vi "ReadU64FromU16FIFO.vi"(1 "FIFO In":refnum<k21>="U16ResponseFIFO") -> (0 "U64":u64)   [LabVIEW 2016]
uses:
  <vilib>/rvi/DataTransferAndStorage/Container/Common/niFpgaContainerExecOnDevCompGetState.vi
  <vilib>/rvi/Emulation/niFpgaEmulationIsFPGAContextNoSignature.vi
  <vilib>/rvi/Emulation/niFpgaSctlEmulationGetInTimedLoop.vi
  <vilib>/rvi/errors/niFpgaSetErrorForExecOnDevCompSimple.vi
  <vilib>/rvi/eio/common/nirviEmuReportErrorAndStop.vi
  <vilib>/rvi/DataTransferAndStorage/Container/Common/niFpgaContainerGetUniqueNameForEmu.vi
  <vilib>/rvi/FIFO/Fifo_Resource/nirvififoEmulationSetSize.vi
  <vilib>/rvi/FIFO/Fifo_Resource/nirviFifoEmulationQueueMgr.vi
  <instcachedir>/0/nirviFifoEmulationQueueMgr_E5CAEC123FF24DC58D834DCA3CDAA9B5.lvgen/nirviFifoEmulationQueueMgr_E5CAEC123FF24DC58D834DCA3CDAA9B5_002.vi
  <vilib>/rvi/FIFO/Fifo_Resource/nirvififoEmulationDetermineInputValidOut.vi
  <vilib>/rvi/FIFO/Fifo_Resource/nirvififoEmulationCreateLock.vi
  <vilib>/rvi/Emulation/niFpgaProcessEmulError.vi
  <vilib>/rvi/FIFO/Fifo_Resource/nirvififoEmulationObtainLock.vi
  <vilib>/rvi/FIFO/Fifo_Resource/nirvififoEmulationReleaseLock.vi
  <vilib>/rvi/occurrence/nirviWaitOnOccurrenceBase.vi
  <vilib>/rvi/errors/nirviReportUnexpectedCaseInternalError.vi
  <vilib>/rvi/errors/nirviReportUnexpectedCaseInternalError (U32).vi
  <vilib>/Utility/error.llb/Clear Errors.vi
  <vilib>/rvi/interface/RandomDataEmulation/niFpgaRandomDataHandleErrors.vi
  <vilib>/rvi/DataTransferAndStorage/Container/XNode/niFpgaContainer.xnode
  <vilib>/rvi/FIFO/Fifo_Resource/niFpgaFifoEmulationRefIn.vi
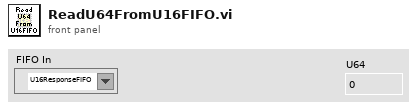
[diagram p1: front panel]
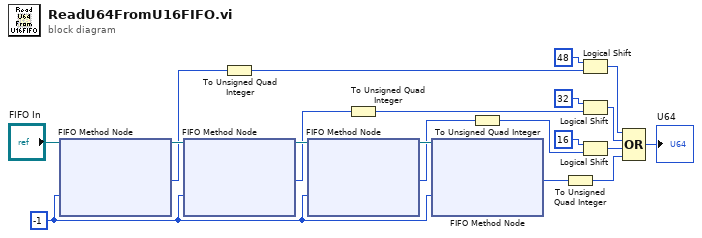
[diagram p0: block diagram]
diagram:
  w13 = -1 ("Timeout")
  n1 = xnode ("FIFO Method Node")("Timeout"=w13, "FIFO In"="FIFO In") -> ("Element"=w15:u16, "FIFO Out"=w19:refnum<k21>)  [unwired: 1 out]
  n2 = xnode ("FIFO Method Node")("Timeout"=w13, "FIFO In"=w19) -> ("Element"=w12:u16, "FIFO Out"=w18:refnum<k21>)  [unwired: 1 out]
  n3 = To Unsigned Quad Integer(1:w15) -> (0:w14:u64)
  n4 = xnode ("FIFO Method Node")("Timeout"=w13, "FIFO In"=w18) -> ("Element"=w11:u16, "FIFO Out"=w17:refnum<k21>)  [unwired: 1 out]
  n5 = To Unsigned Quad Integer(1:w12) -> (0:w9:u64)
  n6 = xnode ("FIFO Method Node")("Timeout"=w13, "FIFO In"=w17) -> ("Element"=w6:u16)  [unwired: 2 out]
  n7 = To Unsigned Quad Integer(1:w11) -> (0:w7:u64)
  n8 = To Unsigned Quad Integer(1:w6) -> (0:w2:u64)
  n9 = Logical Shift(y=i16 48, x=w14) -> (x << y=w5:u64)
  n10 = Logical Shift(y=i16 32, x=w9) -> (x << y=w4:u64)
  n11 = Logical Shift(y=i16 16, x=w7) -> (x << y=w3:u64)
  n12 = Compound Arithmetic op=OR(w5, w4, w3, w2) -> (→"U64":u64)
